vi "KundtsTube.vi"() -> ()   [LabVIEW 2014]
panel:
  out "AC estimate (Vrms)":dbl format="%0.2f"
  in  "Seconds to wait":u32
  in  "stop":bool
  in  "Digitizing Parameters":T1
  out "XY Graph":cluster{"Y":dbl[], "Y":dbl[]}[](graph)
  out "Waveform Graph":dynamicdata(graph)
  in  "Amplitude":dbl
  in  "?":enum32{"Sweep", "Single"}(tab)
  in  "Spacing":enum16{"Logarithmic", "Linear"}(ring)
  in  "# of Points":dbl
  in  "Maximum":dbl
  in  "Minimum":dbl
  in  "Knob":dbl(knob) scale=0.0..20000.0
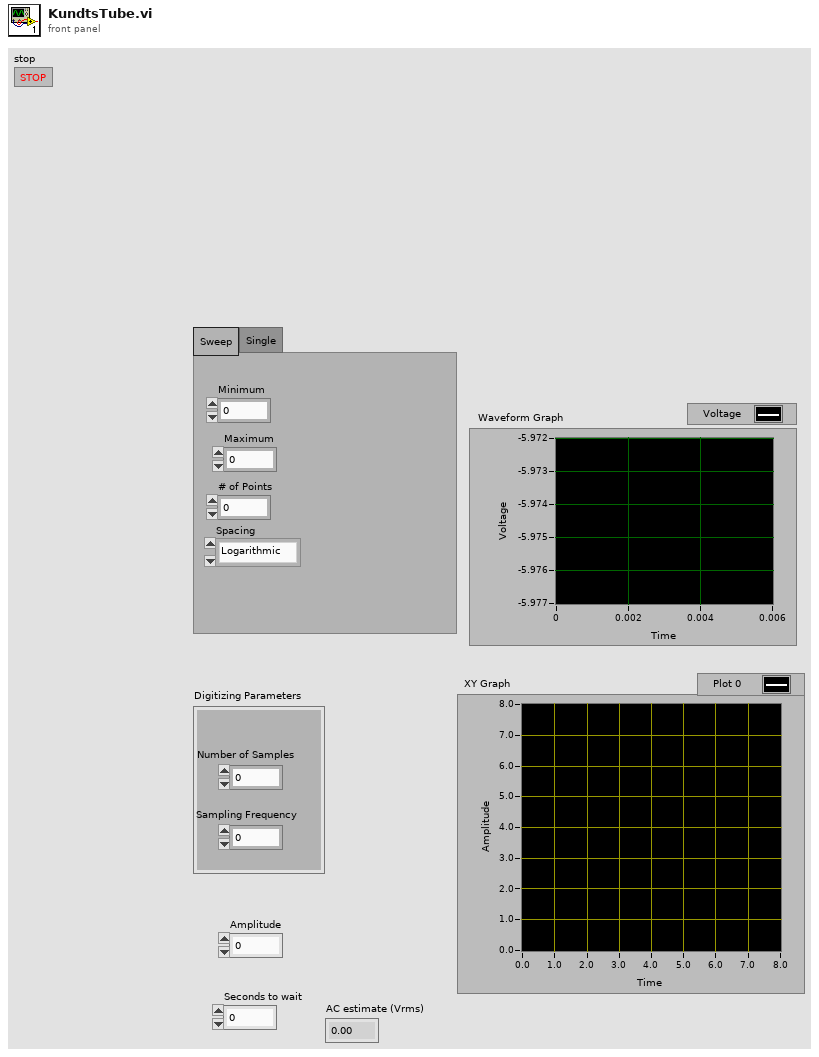
[diagram p1: front panel]
types:
  T1 = cluster{"Number of Samples":dbl, "Sampling Frequency":dbl}
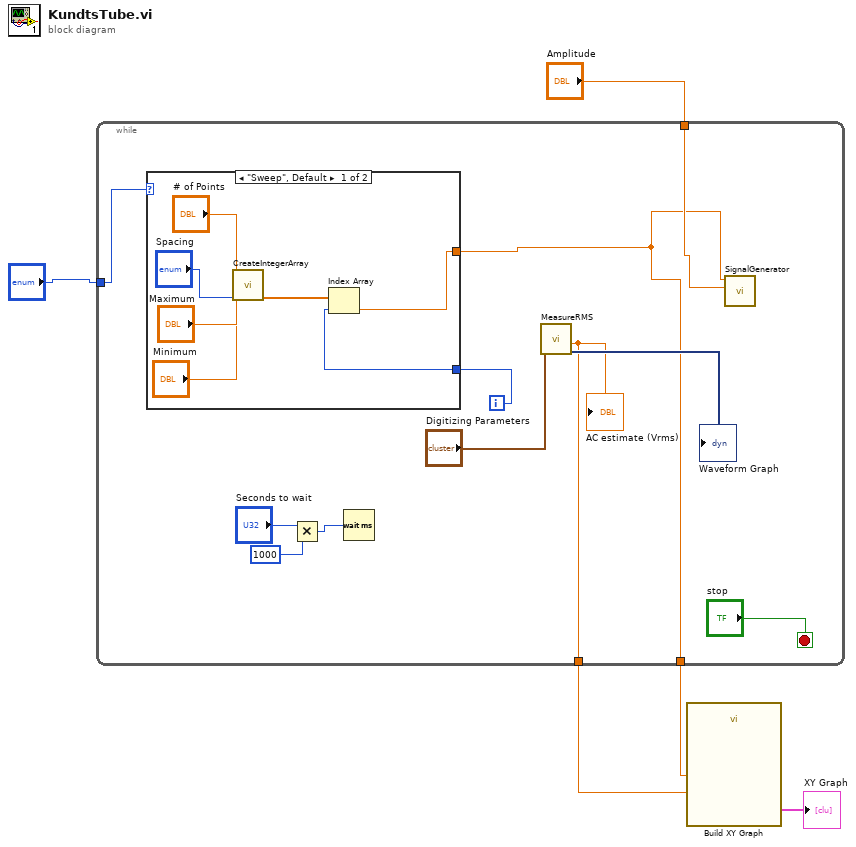
[diagram p0: block diagram]
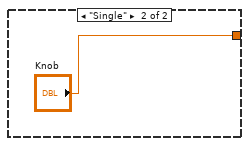
[diagram p2: hidden frame]
diagram:
  n1 = while {
    tunnel: "?" -> [w11]
    tunnel: [w13] -> w3
    tunnel: "Amplitude" -> [w15]
    tunnel: [w6] -> w1
    i -> [w12]
    stop <- "stop" stop-if-true
    n2 = case shown="\"Sweep\", Default" w11 {
      tunnel: [w17 "Knob"] -> w13
      tunnel: w12 -> [w19 _]
      frame "Sweep", Default {
        n3 = call "CreateIntegerArray.vi"("Spacing"="Spacing", "# of Points"="# of Points", "Maximum"="Maximum", "Minimum"="Minimum") -> ("Out"=w18:dbl[])  [unwired: 7 in]
        n4 = Index Array(array=w18, index=w19) -> (element=w17:dbl)
      }
      frame "Single" {
      }
    }
    n5 = Multiply(x="Seconds to wait", y=u32 1000) -> (x*y=w7:u32)
    n6 = Wait (ms)(milliseconds to wait=w7) -> ()  [unwired: 1 out]
    n7 = call "MeasureRMS.vi"("Digitizing Parameters"="Digitizing Parameters") -> ("Waveform Graph"=→"Waveform Graph":dynamicdata, "AC estimate (Vrms)"=w6:dbl)  [unwired: 8 in, 1 out]
    "AC estimate (Vrms)" <- w6
    n8 = call "SignalGenerator.vi"("Amplitude"=w15, "Frequency"=w13) -> ()  [unwired: 9 in, 1 out]
  }
  n9 = call "Build XY Graph"("Y Input"=w1, "X Input"=w3) -> ("XY Graph"=→"XY Graph":cluster{"X":dbl[], "Y":dbl[]}[])  [unwired: 8 in, 1 out]
